vi "AuMT8852B Set Cached String Attribute.vi"(5 "Value (\"\")":string, 8 "error in (no error)":errorcluster, 10 "Attribute ID":T2, 11 "VISA session":refnum<visa-resource-name>) -> (0 "error out":errorcluster, 3 "VISA session out":refnum<visa-resource-name>)   [LabVIEW 2017]
doc: "Anritsu MT8852B Bluetooth Tester\n\nWrites an attribute value directly into the cache.\n\nINPUTS\nAttribute ID - which attribute is being written.\nValue - value to write into the cache."
uses:
  <instrlib>/aumt8852B/General/Utilities/MT8850 Attribute ID.ctl
  <instrlib>/aumt8852B/General/Utilities/Instrument.llb/Instrument Object Reference.ctl
panel:
  in  "reference":T1
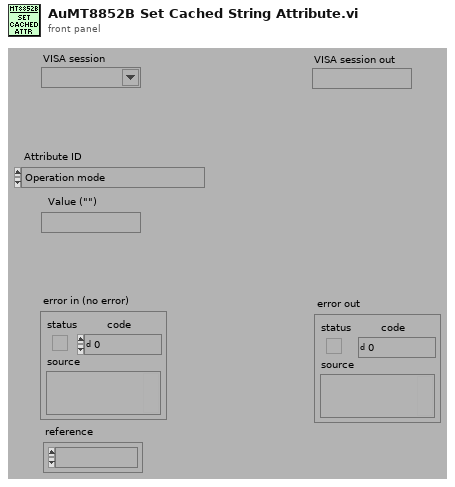
[diagram p1: front panel]
types:
  T1 = typedef "Instrument Object Reference.ctl" = refnum<k1>
  T2 = typedef "MT8850 Attribute ID.ctl" = enum16{"Operation mode", "Selected script", "EUT address source", "EUT Address", "EUT HCI RS232 Baud Rate", "Tester GPIB Address", "Tester RS232 Baud Rate", "Tester Bluetooth Address", "Tester Contrast", "Tester Key Click On", "Tester Modulation Index", "Tester Poll-Null Mode", "Tester Power Range", "Tester RS232 Mode", "Beep on Illegal Entry", "Display User Text", "User Text", "Calibration TX Modulation DAC", "Calibration RX Channel", "Calibration TX Channel", "Calibration TX Power", "Calibration Use TX Table", "Inquiry Request User-friendly Name", "Inquiry Number of Responses", "Inquiry Timeout", "Script Frequency Display", "Script Loop Count", "Script Loop Continuously", "Script Loop Stop on Fail", "Link timeout", "Page timeout", "Filter bandwidth", "SCO air code", "SCO bit position", "SCO input code", "SCO input data", "SCO input sample size", "SCO loopback mode", "SCO packet type", "SCO tone generator", "Tester page scan repetition mode", "Tester follow test mode", "Tester authentication state", "Tester authentication pin code", "Tester authentication pin length"}
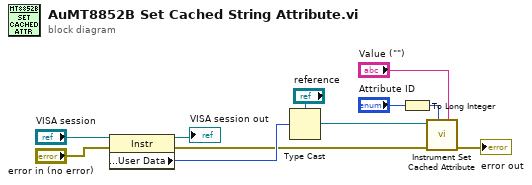
[diagram p0: block diagram]
diagram:
  n1 = property class="Instr"(reference="VISA session", error in="error in (no error)") -> (reference out=→"VISA session out":refnum<visa-resource-name>, error out=w4:errorcluster, "General Settings:User Data"=w7:u32)
  n2 = Type Cast(type="reference", x=w7) -> (*(type *) &x=w5:T1)
  n3 = To Long Integer(number="Attribute ID") -> (32bit integer=w3:i32)
  n4 = call <instrlib>:"Instrument Set Cached Attribute.vi"("Flattened value (\"\")"="Value (\"\")", "Attribute ID"=w3, "error in (no error)"=w4, "reference"=w5) -> ("error out"=→"error out":errorcluster)  [unwired: 6 in, 1 out]
